vi "PicoScope6000ExampleRapidBlockBulkOverlapped.vi"() -> ()   [LabVIEW 2010]
uses:
  shared/PicoBuffers.ctl
  shared/Buffer and Transfer Settings.ctl
  shared/Acquisition Settings.ctl
  shared/Segment Range.ctl
  PicoScope6000Lib/PicoScope6000AnalogChannelSettings.ctl
panel:
  out "Trigger Offsets":cluster{u64, sgl}[](array[cluster]) {"?" format="%#_5p"}
  out "Properties Panel":T1 {"Max Total Capture Time Available (sec)" format="%.3p"; "Sample Frequency" format="%.3p"; "Sample Internal" format="%.3p"; "Max Samples Available" format="%.3p"; "Total Capture Time (sec)" format="%.3p"}
  in  "Trigger Settings":T2={"Trigger Enabled"=FALSE, "Trigger Source"=enum."Channel A", "Trigger Threshold (Volts)"=0.0, "Trigger Direction"=2, "Trigger Delay (samples)"=0, "Auto Trigger Time (ms)"=1000} {"Trigger Direction" items=["Rising"=2, "Falling"=3]}
  in  "Channel A Settings":T3={"Enabled"=TRUE, "Coupling"=1, "Range"=6, "Analogue Offset"=0.0, "Bandwidth"=0} {"Bandwidth" items=["Full", "20 MHz"]; "Range" items=["10 mV", "20 mV", "50 mV", "100 mV", "200 mV", "500 mV", "1 V", "2 V", "5 V", "10 V", "20 V", "50 V ", "100 V"]; "Coupling" items=["AC", "DC 1 MOhm", "DC 50 Ohm"]}
  in  "Write ChA to file":bool
  out "overflow":i16[](array[numeric]) format="%04d"
  in  "Stop Display":bool
  out "Capture Complete":bool
  in  "Run":bool
  in  "Display Buffer Index":i32
  in  "Segment Range":T4={"fromSegmentIndex"=0, "toSegmentIndex"=9} {"toSegmentIndex" format="%.4p"; "fromSegmentIndex" format="%.4p"}
  in  "nSegments":u64=10 format="%.4p"
  out "error out":errorcluster
  in  "Data file":path=path "PicoScopeospaExampleRapidBlock ChA Data"
  in  "Buffer and Transfer Settings":T5={"startIndex"=0, "Samples"=10000000, "Down Sample Ratio"=1, "Down-Sample Mode"=0} {"Down-Sample Mode" items=["None"=0, "Aggregate"=1, "Decimate"=2, "Average"=4]; "Down Sample Ratio" step=1; "Samples" format="%_6p"}
  in  "Acquisition Settings":T6={"preTriggerSamples"=0, "postTriggerSamples"=10000000, "timebase"=5} {"postTriggerSamples" format="%_6p"; "preTriggerSamples" format="%_6p"}
  in  "stop":bool
  out "Analog Channels":cluster{i32, sgl, "Data":dbl[]}[](graph)
  in  "Serial Number":string
  in  "Use Serial Number":bool
  in  "error in (no error)":errorcluster
  # "Bit 0 = ChA"
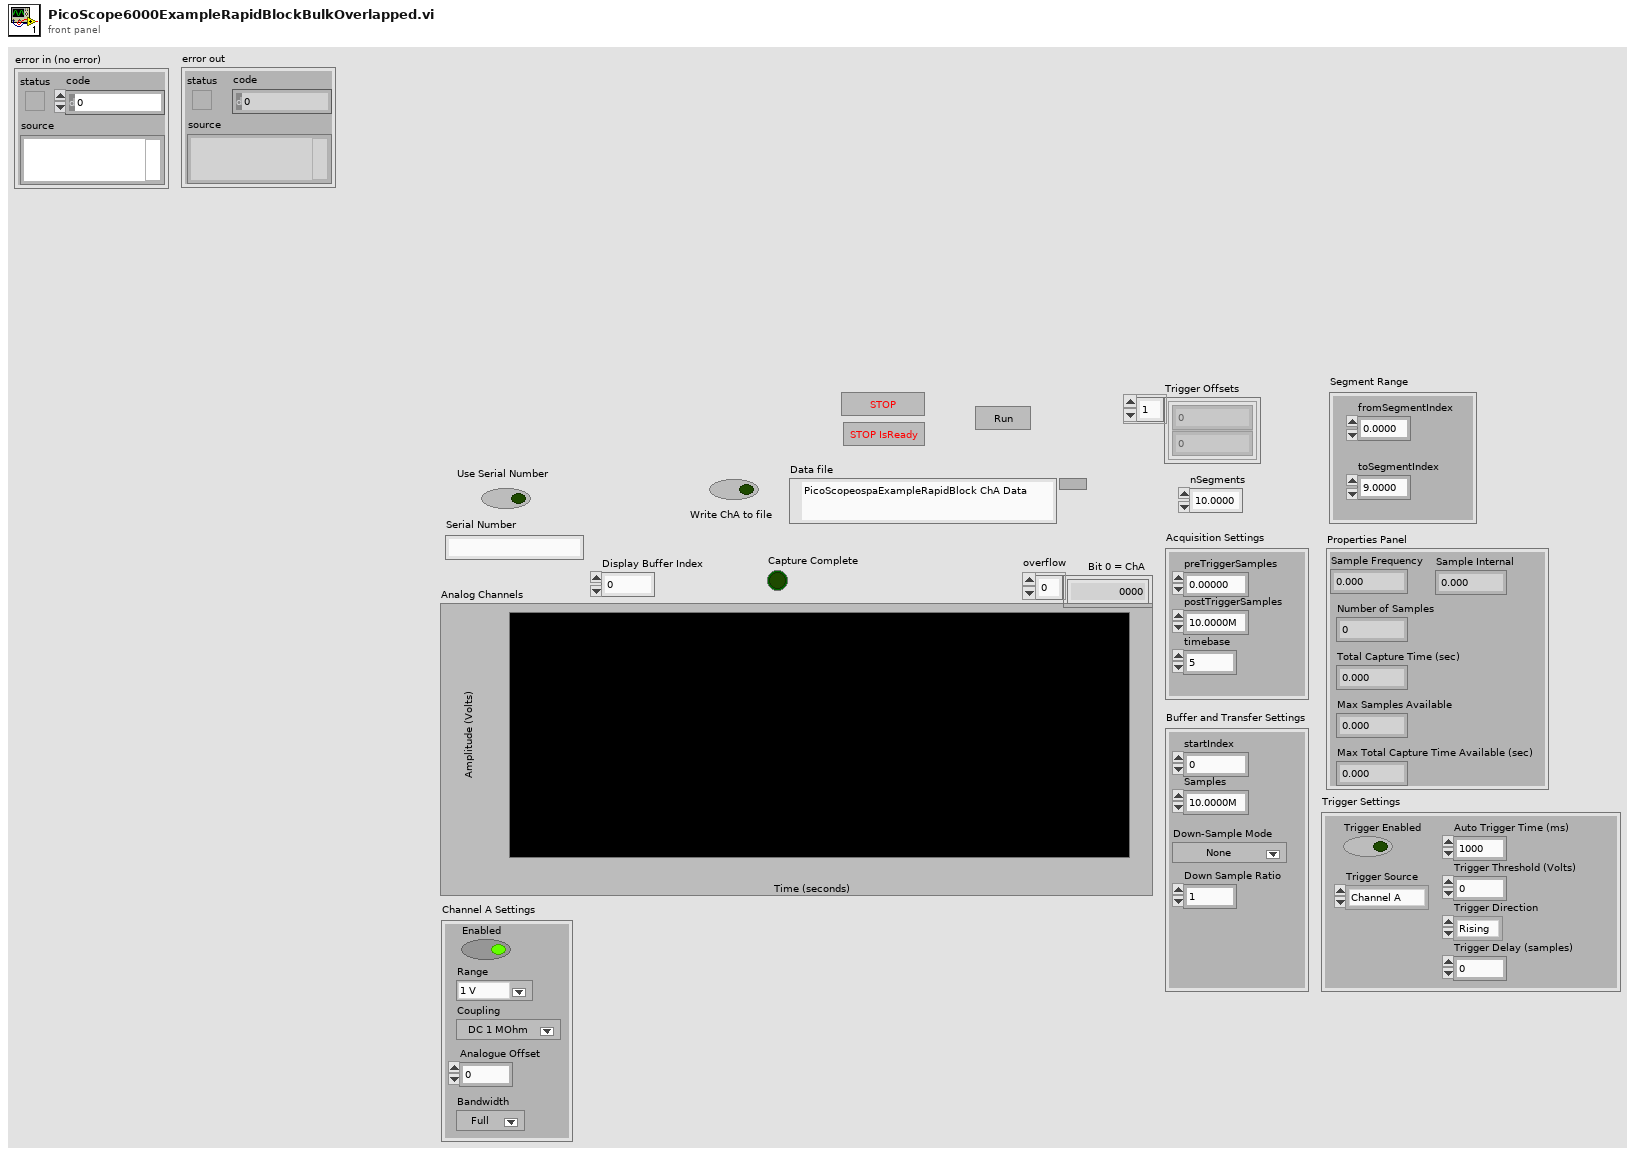
[diagram p1: front panel]
types:
  T1 = cluster{"Sample Frequency":sgl, "Sample Internal":sgl, "maxSamples":u32, "Number of Samples":u32, "Total Capture Time (sec) ":sgl, "Max Total Capture Time Available (sec)":sgl}
  T2 = cluster{"Trigger Enabled":bool, "Trigger Source":enum32{"Channel A", "Channel B", "Channel C", "Channel D", "External", "Aux."}, "Trigger Threshold (Volts)":dbl, "Trigger Direction":u16, "Trigger Delay (samples)":u32, "Auto Trigger Time (ms)":i16}
  T3 = typedef "PicoScope6000AnalogChannelSettings.ctl" = cluster{"Enabled":bool, "Coupling":u32, "Range":u32, "Analogue Offset":sgl, "Bandwidth":u32}
  T4 = typedef "Segment Range.ctl" = cluster{"fromSegmentIndex":u64, "toSegmentIndex":u64}
  T5 = typedef "Buffer and Transfer Settings.ctl" = cluster{"startIndex":u64, "Samples":u64, "Down Sample Ratio":u64, "Down-Sample Mode":u32}
  T6 = typedef "Acquisition Settings.ctl" = cluster{"preTriggerSamples":u64, "postTriggerSamples":u64, "timebase":u32}
  T7 = typedef "PicoBuffers.ctl" = cluster{"Max Buffer Pointers":u64[][][], "Min Buffer Pointers":u64[][][], "StreamingDataInfo":cluster{"Channel":u32, "Down-Sample Mode":u32, "PICO_DATA_TYPE":enum32{"PICO_INT8_T", "PICO_INT16_T", "PICO_INT32_T", "PICO_UINT32_T", "PICO_INT64_T", ""}, "Samples":i32, "bufferIndex":u64, "startIndex":i32, "overflow":i16}[][]}
  T8 = enum16{"open", "open or create", "create or replace", "create", "open (read-only)"}
  T9 = cluster{"Driver Version":string, "USB Version":string, "Hardware":string, "Variant":string, "Batch and Serial":string, "Cal Date":string, "Kernel Version":string, "Digital HW Version":string, "Analogue HW Version":string, "Firmware v1":string, "Firmware v2":string, "Channels":i16}
  T10 = cluster{"Channel A Buffer":i16[], "Channel B Buffer":i16[], "Channel C Buffer":i16[], "Channel D Buffer":i16[], "Channel E Buffer":i16[], "Channel F Buffer":i16[], "Channel G Buffer":i16[], "Channel H Buffer":i16[], "Port 0 Buffer":i16[], "Port 1 Buffer":i16[]}[]
  T11 = cluster{"Channel A Buffer":i16[], "Channel B Buffer":i16[], "Channel C Buffer":i16[], "Channel D Buffer":i16[], "Channel E Buffer":i16[], "Channel F Buffer":i16[], "Channel G Buffer":i16[], "Channel H Buffer":i16[], "Port 0 Buffer":i16[], "Port 1 Buffer":i16[]}
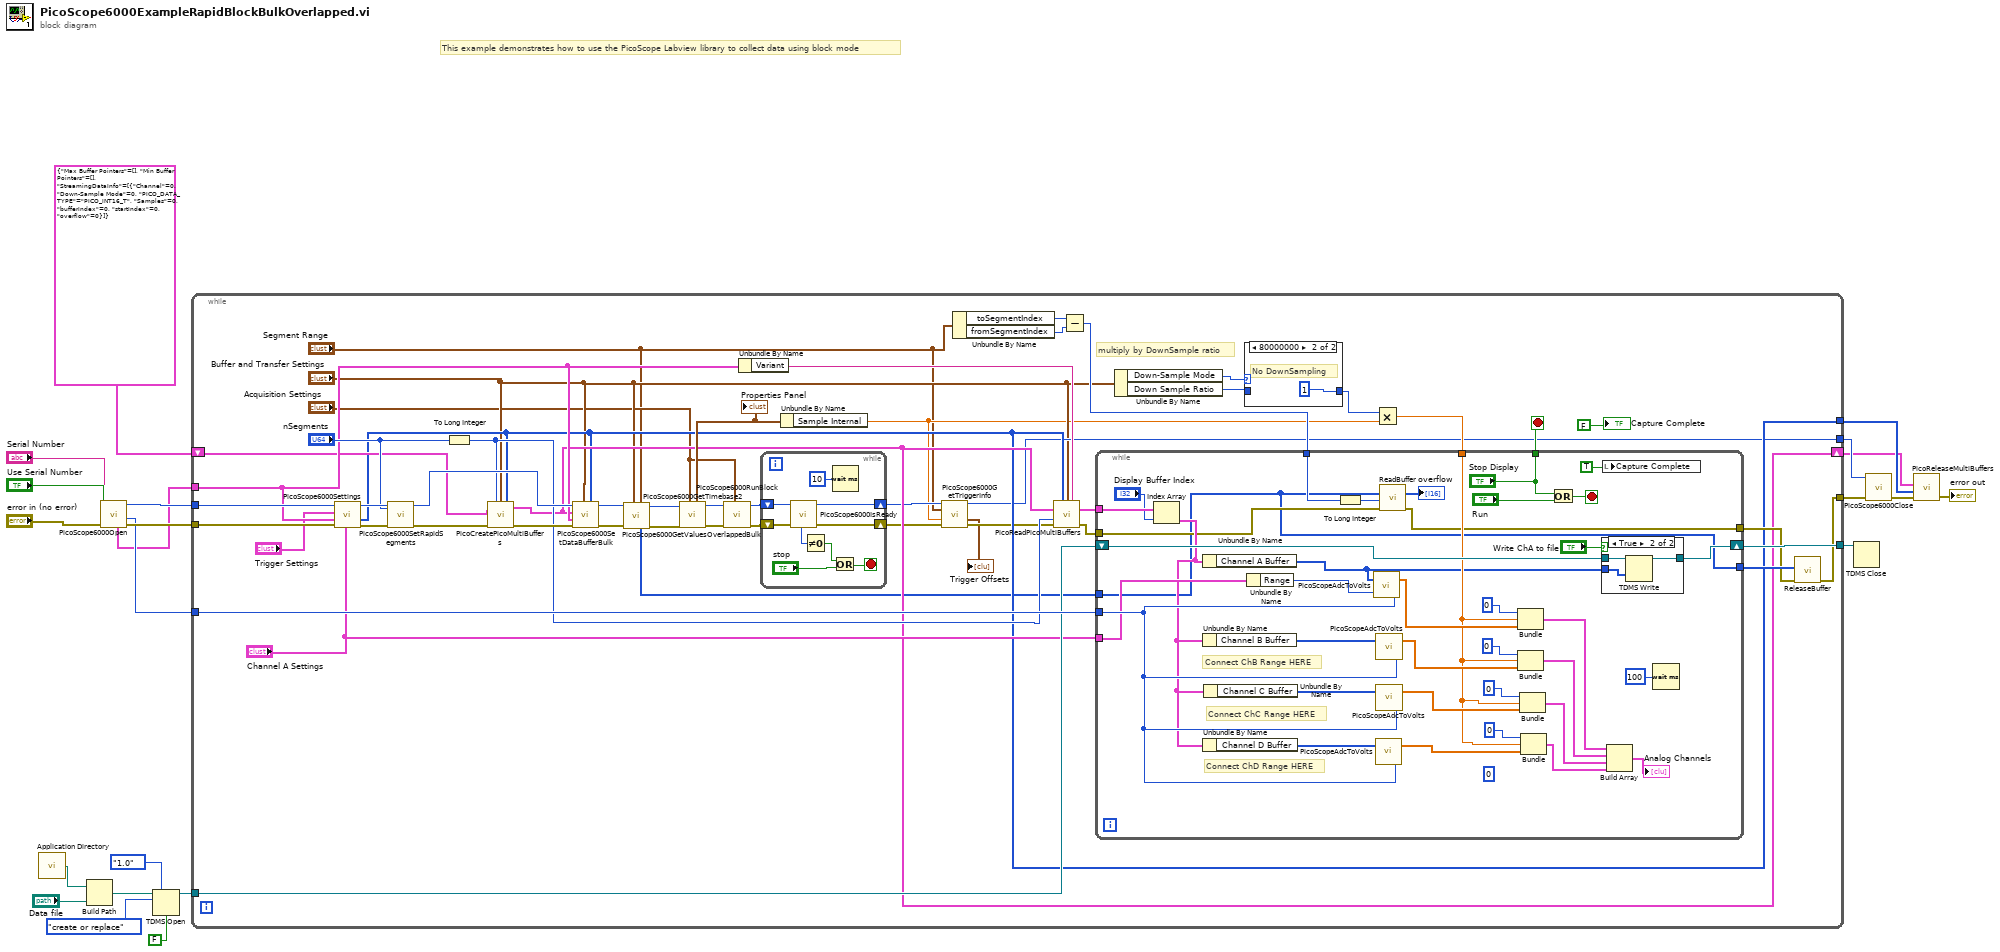
[diagram p0: block diagram]
diagram:
  # "This example demonstrates how to use the PicoScope Labview library to collect data using block mode"
  n1 = call <vilib>:"Application Directory.vi"() -> ("Application Directory"=w7:path)
  n2 = Build Path(base path=w7, name or relative path="Data file") -> (appended path=w8:path)
  n3 = call "PicoScope6000Open.vi"("error in (no error)"="error in (no error)", "Serial Number"="Serial Number", "Use Serial Number"="Use Serial Number") -> ("error out"=w18:errorcluster, "Max Adc value"=w17:i16, "handle"=w19:i16, "Device Info"=w3:T9)  [unwired: 4 in, 1 out]
  n4 = TDMS Open(6:FALSE ("disable buffering? (T)"), 7:enum16{"1.0", "2.0"}."1.0" ("file format version (2.0)"), 10:T8."create or replace" ("operation (0:open)"), 11:w8) -> (3:w5:refnum<k34>)  [unwired: 2 in, 1 out]
  n5 = while {
    tunnel: w3 -> [w41]
    tunnel: w17 -> [w72]
    tunnel: w19 -> [w74]
    tunnel: [w28] -> w14
    tunnel: w18 -> [w73]
    tunnel: [w44] -> w15
    tunnel: [w37] -> w16
    tunnel: [w70] -> w6
    tunnel: w5 -> [w69]
    shift-right: [w39] -> w1
    shift-left: T7 {"Max Buffer Pointers"=[], "Min Buffer Pointers"=[], "StreamingDataInfo"=[[{"Channel"=0, "Down-Sample Mode"=0, "PICO_DATA_TYPE"=enum."PICO_INT16_T", "Samples"=0, "bufferIndex"=0, "startIndex"=0, "overflow"=0}]]} ("Data Pointers") -> [w40]
    stop <- w51 stop-if-true
    # "multiply by DownSample ratio"
    n6 = call "PicoScope6000Settings.vi"("Channel A Settings"="Channel A Settings", "error in"=w73, "Device Info"=w41, "Trigger Settings"="Trigger Settings", "handle in"=w74) -> ("error out"=w68:errorcluster, "Enabled array"=w37:i16[], "handle out"=w67:i16)  [unwired: 4 in]
    n7 = call "PicoScope6000SetRapidSegments.vi"("nSegments"="nSegments", "error in (no error)"=w68, "handle in"=w67) -> ("error out"=w66:errorcluster, "handle out"=w65:i16)  [unwired: 6 in, 1 out]
    n8 = To Long Integer(number="nSegments") -> (32bit integer=w63:i32)
    n9 = call "PicoCreatePicoMultiBuffers.vi"("Number of Buffers"=w63, "Buffer and Transfer Settings"="Buffer and Transfer Settings", "enabled array"=w37, "Data Pointers In"=w40, "error in (no error)"=w66) -> ("Data Pointers"=w39:T7, "error out"=w71:errorcluster)  [unwired: 9 in]
    n10 = call "PicoScope6000SetDataBufferBulk.vi"("enabled array"=w37, "Buffer and Transfer Settings"="Buffer and Transfer Settings", "error in (no error)"=w71, "Device Info"=w41, "Data Pointers In"=w39, "handle in"=w65) -> ("error out"=w36:errorcluster, "handle out"=w35:i16)  [unwired: 4 in]
    n11 = call "PicoScope6000GetValuesOverlappedBulk.vi"("Segment Range"="Segment Range", "Buffer and Transfer Settings"="Buffer and Transfer Settings", "error in (no error)"=w36, "handle in"=w35) -> ("error out"=w34:errorcluster, "handle out"=w33:i16, "overflow"=w32:u64[])  [unwired: 4 in, 1 out]
    n12 = call "PicoScope6000GetTimebase2.vi"("Acquisition Settings"="Acquisition Settings", "error in (no error)"=w34, "handle in"=w33) -> ("error out"=w55:errorcluster, "handle out"=w56:i16, "Properties Panel"=w59:T1)  [unwired: 6 in]
    "Properties Panel" <- w59
    n13 = call "PicoScope6000RunBlock.vi"("Acquisition Settings"="Acquisition Settings", "error in (no error)"=w55, "handle in"=w56) -> ("error out"=w54:errorcluster, "handle out"=w53:i16)  [unwired: 5 in, 2 out]
    n14 = Unbundle By Name(w41) -> ("Variant"=w49:string)
    n15 = while {
      shift-right: [w124] -> w31
      shift-left: w54 -> [w125]
      shift-right: [w123] -> w29
      shift-left: w53 -> [w122]
      stop <- w120 stop-if-true
      n16 = call "PicoScope6000IsReady.vi"("error in (no error)"=w125, "handle in"=w122) -> ("error out"=w124:errorcluster, "handle out"=w123:i16, "ready"=w121:i16)  [unwired: 7 in]
      n17 = Not Equal To 0?(x=w121) -> (x != 0?=w119:bool)
      n18 = Or(x=w119, y="stop") -> (x .or. y?=w120:bool)
      n19 = Wait (ms)(milliseconds to wait=u32 10) -> ()  [unwired: 1 out]
    }
    n20 = Unbundle By Name(w59) -> ("Sample Internal"=w25:sgl)
    n21 = call "PicoScope6000GetTriggerInfo.vi"("handle in"=w29, "Segment Range"="Segment Range", "Sample Rate"=w25, "error in"=w31) -> ("handle out"=w28:i16, "Trigger Offsets"=→"Trigger Offsets":cluster{u64, sgl}[], "error out"=w30:errorcluster)  [unwired: 8 in, 1 out]
    n22 = Unbundle By Name("Segment Range") -> ("toSegmentIndex"=w47:u64, "fromSegmentIndex"=w46:u64)
    n23 = call "PicoReadPicoMultiBuffers.vi"("enabled array"=w37, "Buffer and Transfer Settings"="Buffer and Transfer Settings", "Variant"=w49, "Data Pointers"=w39, "No of Buffers"=w63, "error in (no error)"=w30) -> ("MultiBuffers (Max or non-aggregated)"=w62:T10, "error out"=w52:errorcluster)  [unwired: 7 in, 1 out]
    n24 = Subtract(x=w47, y=w46) -> (x-y=w48:u64)
    n25 = Unbundle By Name("Buffer and Transfer Settings") -> ("Down-Sample Mode"=w60:u32, "Down Sample Ratio"=w61:u64)
    n26 = case shown="80000000" w60 {
      tunnel: [w126 u64 1 ("Down Sample Ratio")] -> w57
      tunnel: w61 -> [w126 _]
      frame Default {
      }
      frame -2147483648 {
        # "No DownSampling"
      }
    }
    n27 = Multiply(x=w57, y=w25) -> (x*y=w58:sgl)
    n28 = while {
      tunnel: w72 -> [w112]
      tunnel: "Channel A Settings" -> [w111]
      tunnel: w62 -> [w91]
      tunnel: w58 -> [w90]
      shift-right: [w110] -> w70
      shift-left: w69 -> [w109]
      tunnel: [w80] -> w43
      tunnel: w52 -> [w81]
      tunnel: ["Stop Display"] -> w51
      tunnel: w32 -> [w76]
      tunnel: w48 -> [w77]
      tunnel: [w76] -> w45
      stop <- w84 stop-if-true
      (unwired) 0
      # "Connect ChD Range HERE"
      # "Connect ChC Range HERE"
      # "Connect ChB Range HERE"
      n29 = Index Array(array=w91, index="Display Buffer Index") -> (element=w89:T11)
      n30 = Unbundle By Name(w89) -> ("Channel A Buffer"=w88:i16[])
      n31 = Unbundle By Name(w89) -> ("Channel B Buffer"=w105:i16[])
      n32 = Unbundle By Name(w89) -> ("Channel D Buffer"=w99:i16[])
      n33 = Unbundle By Name(w89) -> ("Channel C Buffer"=w100:i16[])
      n34 = Unbundle By Name(w111) -> ("Range"=w107:u32)
      n35 = To Long Integer(number=w77) -> (32bit integer=w78:i32)
      n36 = call "PicoScopeAdcToVolts.vi"("Max_adc"=w112, "Range Index"=w107, "Data"=w88) -> ("Data"=w92:dbl[])
      n37 = call "PicoScopeAdcToVolts.vi"("Max_adc"=w112, "Data"=w99) -> ("Data"=w95:dbl[])  [unwired: 1 in]
      n38 = call "PicoScopeAdcToVolts.vi"("Max_adc"=w112, "Data"=w105) -> ("Data"=w104:dbl[])  [unwired: 1 in]
      n39 = call "PicoScopeAdcToVolts.vi"("Max_adc"=w112, "Data"=w100) -> ("Data"=w96:dbl[])  [unwired: 1 in]
      n40 = call "ReadBuffer.vi"("Pointer and BufferSize"=w76, "Buffer size"=w78, "error in (no error)"=w81) -> ("Output Array"=→"overflow":i16[], "error out"=w80:errorcluster)  [unwired: 11 in]
      n41 = Bundle(0, w90, "Data"=w92) -> (w103:cluster{i32, sgl, "Data":dbl[]})  [unwired: 1 in]
      n42 = Bundle(0, w90, "Data"=w104) -> (w102:cluster{i32, sgl, "Data":dbl[]})  [unwired: 1 in]
      n43 = Bundle(0, w90, "Data"=w96) -> (w94:cluster{i32, sgl, "Data":dbl[]})  [unwired: 1 in]
      n44 = Bundle(0, w90, "Data"=w95) -> (w93:cluster{i32, sgl, "Data":dbl[]})  [unwired: 1 in]
      n45 = Or(x="Stop Display", y="Run") -> (x .or. y?=w84:bool)
      n46 = case shown="True" "Write ChA to file" {
        tunnel: [w113 w116] -> w110
        tunnel: w109 -> [w113 w115]
        tunnel: w88 -> [_ w114]
        frame False {
        }
        frame True {
          n47 = TDMS Write(0:w115, 9:w114) -> (4:w116:refnum<k34>)  [unwired: 4 in, 3 out]
        }
      }
      n48 = local write "Capture Complete"(TRUE ("Capture Complete")) -> ()
      n49 = Build Array(w103, w102, w94, w93) -> (→"Analog Channels":cluster{i32, sgl, "Data":dbl[]}[])
      n50 = Wait (ms)(milliseconds to wait=u32 100) -> ()  [unwired: 1 out]
    }
    n51 = call "ReleaseBuffer.vi"("error in (no error)"=w43, "Pointer and BufferSize"=w45) -> ("error out"=w44:errorcluster)  [unwired: 9 in]
    "Capture Complete" <- FALSE ("Capture Complete")
  }
  n52 = TDMS Close(11:w6) -> ()  [unwired: 1 in, 2 out]
  n53 = call "PicoScope6000Close.vi"("error in (no error)"=w15, "handle"=w14) -> ("error out"=w13:errorcluster)  [unwired: 8 in, 1 out]
  n54 = call "PicoReleaseMultiBuffers.vi"("error in (no error)"=w13, "Enabled array"=w16, "Data Pointers"=w1) -> ("error out"=→"error out":errorcluster)  [unwired: 7 in, 1 out]
